vi "myPID.vi"(4 "Output limits":cluster{"high":dbl, "low":dbl}, 5 "manual input":dbl, 6 "PID gains":T1, 7 "manual/auto":bool, 8 "dt (s)":dbl, 9 "PID data in":dbl[](array[numeric]), 10 "setpoint":dbl, 11 "process variable":dbl) -> (1 "PID data out":dbl[](array[numeric]), 3 "Output":dbl)   [LabVIEW 2020]
panel:
  in  "Anti-windup on":bool
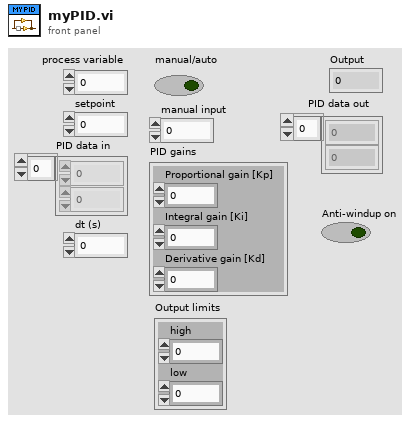
[diagram p1: front panel]
types:
  T1 = cluster{"Proportional gain [Kp]":dbl, "Integral gain [Ki]":dbl, "Derivative gain [Kd]":dbl}
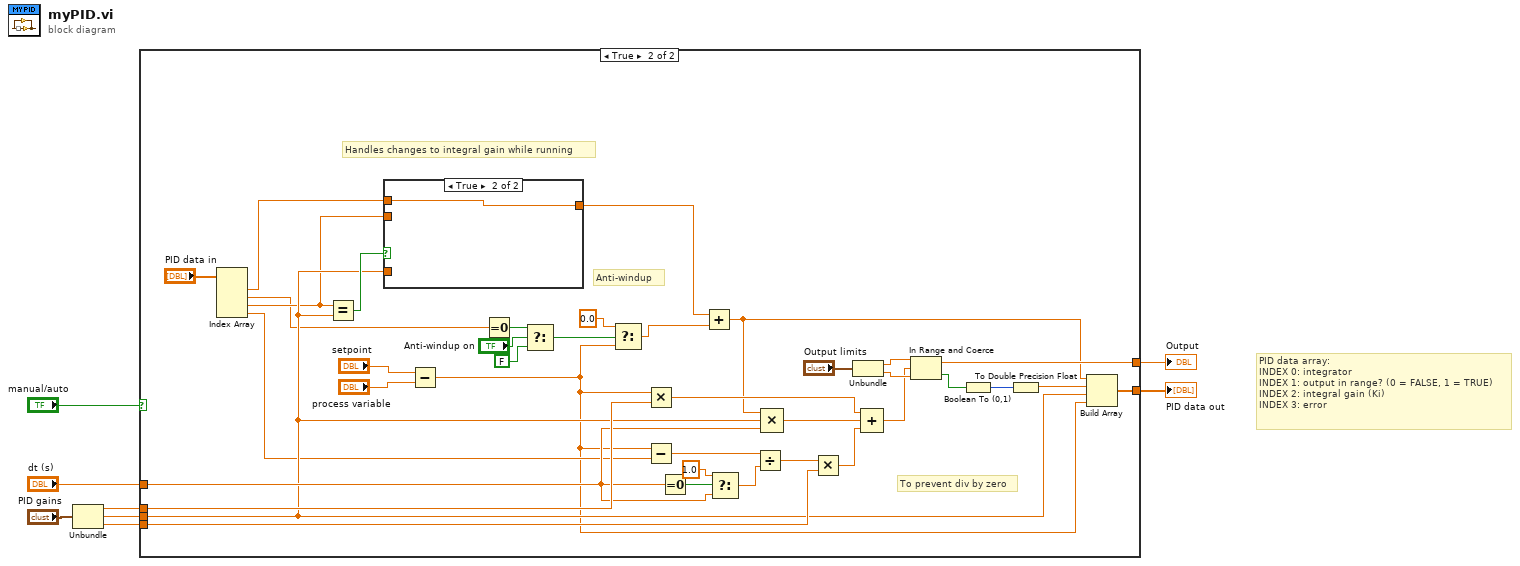
[diagram p0: block diagram]
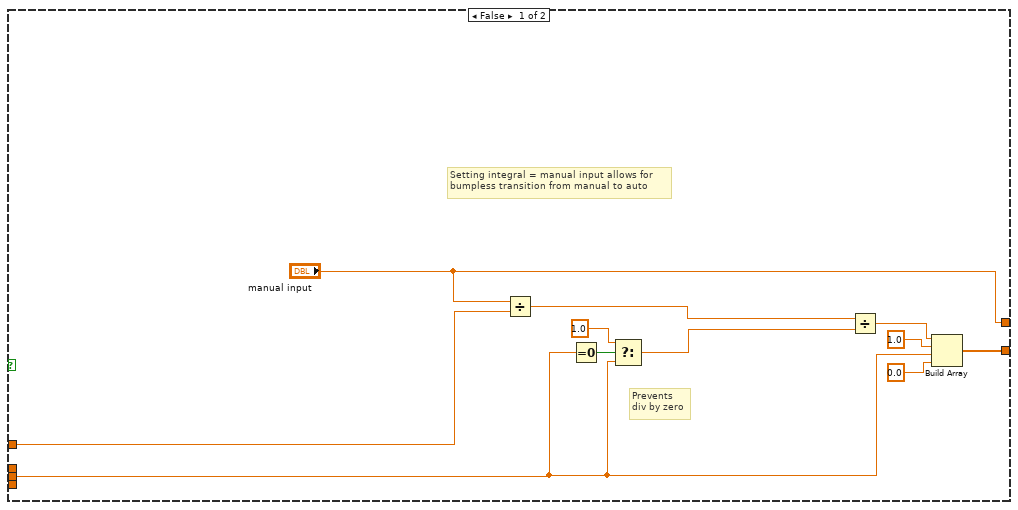
[diagram p2: hidden frame]
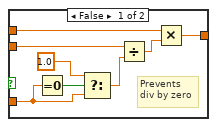
[diagram p3: hidden frame]
diagram:
  # "PID data array:\nINDEX 0: integrator\nINDEX 1: output in range? (0 = FALSE, 1 = TRUE)\nINDEX 2: integral gain (Ki)\nINDEX 3: error"
  n1 = Unbundle("PID gains") -> ("Proportional gain [Kp]"=w5:dbl, "Integral gain [Ki]"=w4:dbl, "Derivative gain [Kd]"=w1:dbl)
  n2 = case shown="True" "manual/auto" {
    tunnel: ["manual input" w57] -> w8
    tunnel: [w12 w50] -> w2
    tunnel: w5 -> [_ w51]
    tunnel: w4 -> [w11 w32]
    tunnel: "dt (s)" -> [w17 w38]
    tunnel: w1 -> [_ w43]
    frame False {
      # "Setting integral = manual input allows for\nbumpless transition from manual to auto"
      # "Prevents\ndiv by zero"
      n3 = Divide(x="manual input", y=w17) -> (x/y=w19:dbl)
      n4 = Equal To 0?(x=w11) -> (x = 0?=w15:bool)
      n5 = Select(t=1.0, s=w15, f=w11) -> (s? t:f=w14:dbl)
      n6 = Divide(x=w19, y=w14) -> (x/y=w13:dbl)
      n7 = Build Array(w13, 1.0 ("element"), w11, 0.0 ("element")) -> (w12:dbl[])
    }
    frame True {
      # "Anti-windup"
      # "To prevent div by zero"
      # "Handles changes to integral gain while running"
      n8 = Index Array(array="PID data in") -> (element #1=w45:dbl, element #2=w28:dbl, element #3=w29:dbl, element #4=w30:dbl)  [unwired: 4 in]
      n9 = Equal?(x=w29, y=w32) -> (x = y?=w48:bool)
      n10 = case shown="True" w48 {
        tunnel: w45 -> [w65 w66]
        tunnel: [w64 w66] -> w35
        tunnel: w29 -> [w63 _]
        tunnel: w32 -> [w60 _]
        frame False {
          # "Prevents\ndiv by zero"
          n11 = Equal To 0?(x=w60) -> (x = 0?=w61:bool)
          n12 = Select(t=1.0, s=w61, f=w60) -> (s? t:f=w62:dbl)
          n13 = Divide(x=w63, y=w62) -> (x/y=w58:dbl)
          n14 = Multiply(x=w65, y=w58) -> (x*y=w64:dbl)
        }
        frame True {
        }
      }
      n15 = Subtract(x="setpoint", y="process variable") -> (x-y=w21:dbl)
      n16 = Equal To 0?(x=w28) -> (x = 0?=w27:bool)
      n17 = Select(t=w27, s="Anti-windup on", f=FALSE) -> (s? t:f=w26:bool)
      n18 = Select(t=0.0, s=w26, f=w21) -> (s? t:f=w22:dbl)
      n19 = Multiply(x=w21, y=w51) -> (x*y=w40:dbl)
      n20 = Subtract(x=w21, y=w30) -> (x-y=w46:dbl)
      n21 = Equal To 0?(x=w38) -> (x = 0?=w39:bool)
      n22 = Add(x=w35, y=w22) -> (x+y=w23:dbl)
      n23 = Select(t=1.0, s=w39, f=w38) -> (s? t:f=w37:dbl)
      n24 = Divide(x=w46, y=w37) -> (x/y=w44:dbl)
      n25 = Compound Arithmetic op=MULTIPLY(w23, w32, w38) -> (w47:dbl)
      n26 = Multiply(x=w44, y=w43) -> (x*y=w41:dbl)
      n27 = Unbundle("Output limits") -> ("high"=w55:dbl, "low"=w54:dbl)
      n28 = Compound Arithmetic op=ADD(w40, w47, w41) -> (w42:dbl)
      n29 = In Range and Coerce(upper limit=w55, x=w42, lower limit=w54) -> (coerced(x)=w57:dbl, In Range?=w34:bool)
      n30 = Boolean To (0,1)(Boolean=w34) -> (0, 1=w33:i16)
      n31 = To Double Precision Float(number=w33) -> (double precision float=w31:dbl)
      n32 = Build Array(w23, w31, w32, w21) -> (w50:dbl[])
    }
  }
  "Output" <- w8
  "PID data out" <- w2
